vi "Sort Properties by Name.vi"(8 "error in (no error)":errorcluster, 11 "properties":refnum<k24>[](array[refnum])) -> (0 "error out":errorcluster, 3 "sorted properties":refnum<k24>[](array[refnum]))   [LabVIEW 2017, in "SLSC Switch Import Unit Tests.lvclass"]
uses:
  SLSC Switch Import Unit Tests.lvclass
  NationalInstruments.VeriStand.SystemStorage
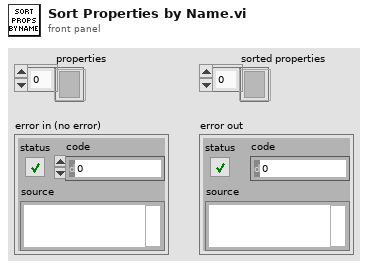
[diagram p1: front panel]
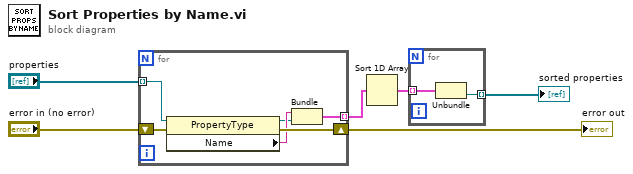
[diagram p0: block diagram]
diagram:
  n1 = for {
    shift-right: [w11] -> w1
    shift-left: "error in (no error)" -> [w10]
    tunnel: "properties" -> [w12] mode=indexing
    tunnel: [w9] -> w4 mode=indexing
    n2 = property class="PropertyType"(reference=w12, error in=w10) -> (reference out=w7:refnum<k24>, error out=w11:errorcluster, "Name"=w8:string)
    n3 = Bundle("Name"=w8, w7) -> (w9:cluster{"Name":string, refnum<k24>})  [unwired: 1 in]
  }
  "error out" <- w1
  n4 = Sort 1D Array(array=w4) -> (sorted array=w3:cluster{"Name":string, refnum<k24>}[])
  n5 = for {
    tunnel: w3 -> [w14] mode=indexing
    tunnel: [w13] -> w2 mode=indexing
    n6 = Unbundle(w14) -> (w13:refnum<k24>)  [unwired: 1 out]
  }
  "sorted properties" <- w2
